vi "Transfer_Chunk_U16_IMG_to_Str.vi"(0 "[IN] U16 Pixel Img":u16[][](array[numeric]), 1 "[IN] # of chunk":i32, 2 "[IN] # rows single transfer":i32, 3 "[IN] # rows last transfer":i32, 4 "[IN] Use remained rows":bool) -> (5 "[OUT] Converted String":string)   [LabVIEW 2020]
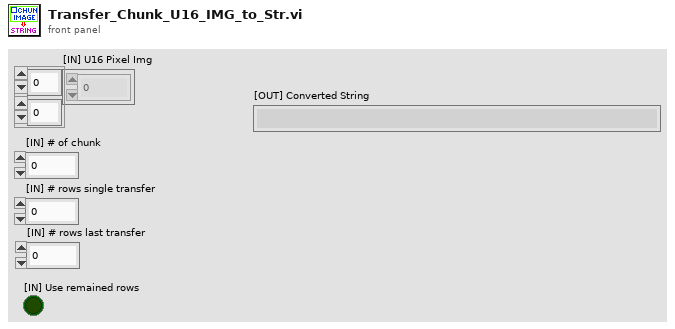
[diagram p1: front panel]
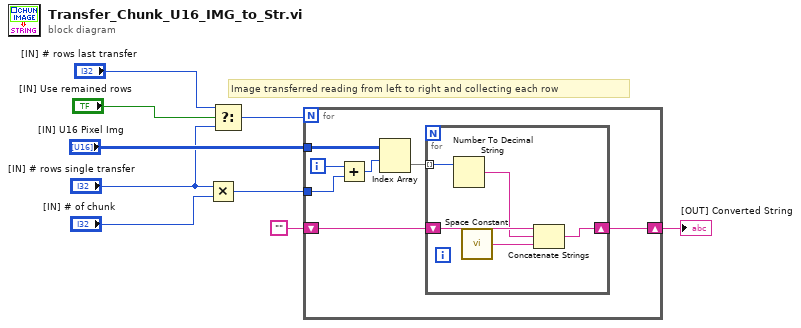
[diagram p0: block diagram]
diagram:
  # "Image transferred reading from left to right and collecting each row"
  n1 = Multiply(x="[IN] # rows single transfer", y="[IN] # of chunk") -> (x*y=w5:i32)
  n2 = Select(t="[IN] # rows last transfer", s="[IN] Use remained rows", f="[IN] # rows single transfer") -> (s? t:f=w2:i32)
  n3 = for {
    N: w2 -> [_]
    tunnel: "[IN] U16 Pixel Img" -> [w16]
    shift-right: [w14] -> w7
    shift-left: "" -> [w15]
    tunnel: w5 -> [w11]
    i -> [w12]
    n4 = Add(x=w12, y=w11) -> (x+y=w10:i32)
    n5 = Index Array(array=w16, index (row)=w10) -> (element=w13:u16[])  [unwired: 1 in]
    n6 = for {
      tunnel: w13 -> [w21] mode=indexing
      shift-right: [w17] -> w14
      shift-left: w15 -> [w20]
      n7 = Number To Decimal String(number=w21) -> (decimal integer string=w19:string)  [unwired: 1 in]
      n8 = call <vilib>:"Space Constant.vi"() -> ("String"=w18:string)
      n9 = Concatenate Strings(w20, w19, w18) -> (w17:string)
    }
  }
  "[OUT] Converted String" <- w7
